vi "Event Trigger.vi"(11 "Boolean":bool=TRUE) -> (2 "State Passthrough":bool, 3 "Event Trigger":bool)   [LabVIEW 2016]
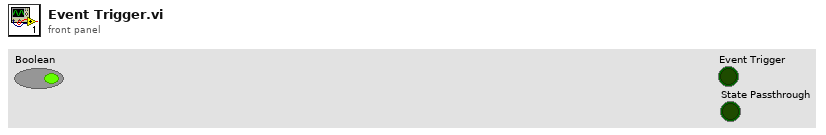
[diagram p1: front panel]
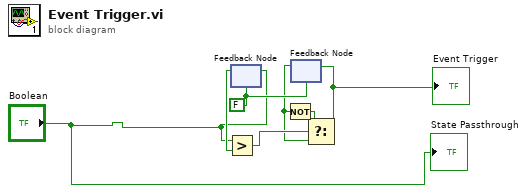
[diagram p0: block diagram]
diagram:
  w5 = FALSE ("Boolean")
  n1 = feedback-in #1("Boolean") -> ()
  n2 = feedback #1(w5) -> (w7:bool)
  n3 = Greater?(x="Boolean", y=w7) -> (0:w6:bool)
  n4 = feedback #2(w5) -> (w4:bool)
  n5 = Not(x=w4) -> (.not. x?=w3:bool)
  n6 = Select(t=w3, s=w6, f=w4) -> (s? t:f=w2:bool)
  "Event Trigger" <- w2
  n7 = feedback-in #2(w2) -> ()
  "State Passthrough" <- "Boolean"
